vi "Lab16.vi"() -> ()   [LabVIEW 2022 SP3]
uses:
  <vilib>/DAQmx/create/channels.llb/DAQmx Create Channel (CO-Pulse Generation-Ticks).vi
  <vilib>/DAQmx/configure/timing.llb/DAQmx Timing (Implicit).vi
  <resource>/objmgr/daqmx.rc
panel:
  in  "Signal Out":tag
  in  "counter":tag
  in  "Signal In":tag="OnboardClock"
  in  "stop":bool
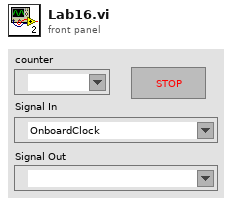
[diagram p1: front panel]
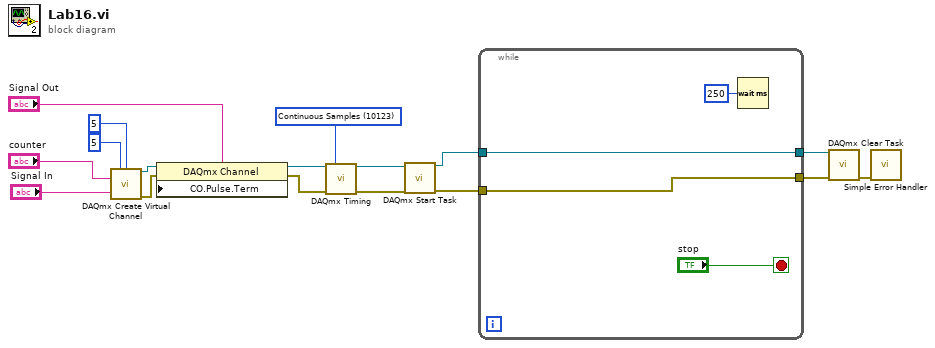
[diagram p0: block diagram]
diagram:
  w1 = 10123 items=["Finite Samples"=10178, "Continuous Samples"=10123, "Hardware Timed Single Point"=12522] ("sample mode")
  n1 = call-poly <vilib>:"DAQmx Create Virtual Channel.vi"("high ticks"=u32 5, "low ticks"=u32 5, "counter"="counter", "source of ticks"="Signal In") -> ("task out"=w12:refnum<k21>, "error out"=w11:errorcluster)  [unwired: 10 in]
  n2 = property class="DAQmx Channel"(reference=w12, error in=w11, "CO.Pulse.Term"="Signal Out") -> (reference out=w9:refnum<k21>, error out=w8:errorcluster)
  n3 = call-poly <vilib>:"DAQmx Timing.vi"("task/channels in"=w9, "sample mode"=w1, "error in"=w8) -> ("task out"=w7:refnum<k21>, "error out"=w6:errorcluster)  [unwired: 11 in]
  n4 = call <vilib>:"DAQmx Start Task.vi"("task/channels in"=w7, "error in"=w6) -> ("task out"=w5:refnum<k21>, "error out"=w4:errorcluster)  [unwired: 12 in]
  n5 = while {
    tunnel: [w21] -> w3
    tunnel: w5 -> [w21]
    tunnel: [w20] -> w2
    tunnel: w4 -> [w20]
    stop <- "stop" stop-if-true
    n6 = Wait (ms)(milliseconds to wait=u32 250) -> ()  [unwired: 1 out]
  }
  n7 = call <vilib>:"DAQmx Clear Task.vi"("task in"=w3, "error in"=w2) -> ("error out"=w17:errorcluster)  [unwired: 13 in]
  n8 = call <vilib>:"Simple Error Handler.vi"("error in (no error)"=w17) -> ()  [unwired: 4 in, 5 out]
